vi "Close.vi"(8 "error in (no error)":errorcluster, 11 "dotNET SSL Listener in":refnum<class "dotNET SSL Listener.lvclass">) -> (0 "error out":errorcluster)   [LabVIEW 2013, in "dotNET SSL Socket.lvlib" / "dotNET SSL Listener.lvclass"]
uses:
  dotNET SSL Listener.lvclass
  dotNET SSL Listener.lvclass/dotNET SSL Listener.ctl
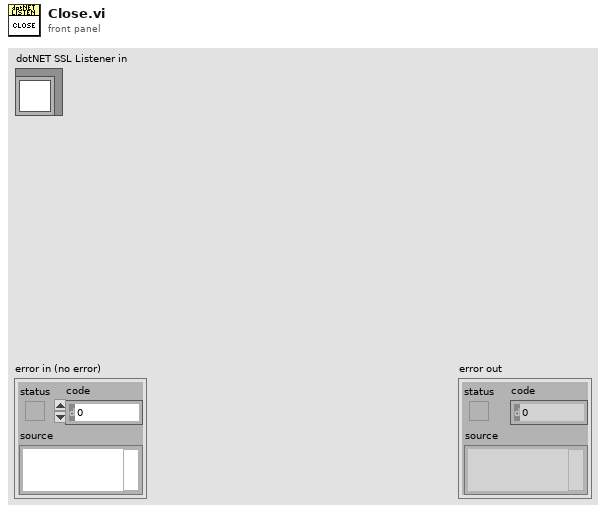
[diagram p1: front panel]
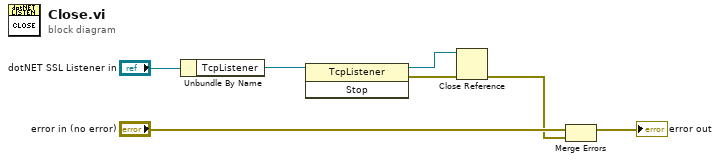
[diagram p0: block diagram]
diagram:
  n1 = Unbundle By Name("dotNET SSL Listener in") -> ("TcpListener"=w5:refnum<k24>)
  n2 = invoke class="TcpListener" method="Stop"(reference=w5) -> (reference out=w1:refnum<k24>, error out=w3:errorcluster)  [unwired: 2 in, 1 out]
  n3 = Close Reference(reference=w1, error in (no error)=w3) -> (error out=w2:errorcluster)
  n4 = Merge Errors("error in (no error)", w2) -> (→"error out":errorcluster)
